vi "svx_Polar_Pixels.vi"() -> (0 "output cluster":T1)   [LabVIEW 2017, in "SVX Polar Plot.xctl"]
uses:
  <vilib>/addons/_XControls/Polar Plot/SVX Polar Plot.xctl
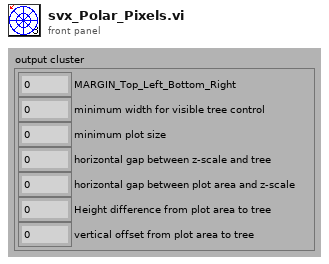
[diagram p1: front panel]
types:
  T1 = cluster{"MARGIN_Top_Left_Bottom_Right":u32, "minimum width for visible tree control":u32, "minimum plot size":u32, "horizontal gap between z-scale and tree":i32, "horizontal gap between plot area and z-scale":i32, "Height difference from plot area to tree":u32, "vertical offset from plot area to tree":u32}
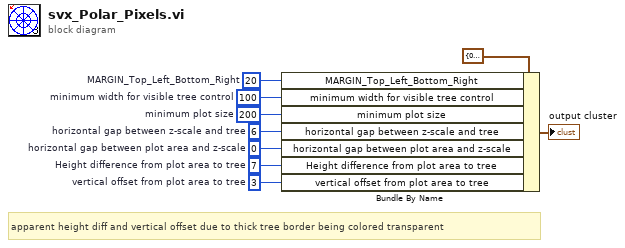
[diagram p0: block diagram]
diagram:
  w7 = u32 200  # minimum plot size
  w5 = 0  # horizontal gap between plot area and z-scale
  w6 = 6  # horizontal gap between z-scale and tree
  w8 = u32 100  # minimum width for visible tree control
  w3 = u32 3  # vertical offset from plot area to tree
  w4 = u32 7  # Height difference from plot area to tree
  w9 = u32 20  # MARGIN_Top_Left_Bottom_Right
  # "apparent height diff and vertical offset due to thick tree border being colored transparent"
  n1 = Bundle By Name(cluster=T1 {"MARGIN_Top_Left_Bottom_Right"=0, "minimum width for visible tree control"=0, "minimum plot size"=0, "horizontal gap between z-scale and tree"=0, "horizontal gap between plot area and z-scale"=0, "Height difference from plot area to tree"=0, "vertical offset from plot area to tree"=0}, "MARGIN_Top_Left_Bottom_Right"=w9, "minimum width for visible tree control"=w8, "minimum plot size"=w7, "horizontal gap between z-scale and tree"=w6, "horizontal gap between plot area and z-scale"=w5, "Height difference from plot area to tree"=w4, "vertical offset from plot area to tree"=w3) -> (→"output cluster":T1)
